vi "Read CellData.vi"(8 "error in":errorcluster, 11 "PAS Data in":refnum<class "PAS Data.lvclass">) -> (0 "error out":errorcluster, 2 "CellData":refnum<class "PAS Cell Data.lvclass">[](array[class]), 3 "PAS Data out":refnum<class "PAS Data.lvclass">)   [LabVIEW 2015, in "PAS Data.lvclass"]
doc: "Retrieve the data associated with the given cell."
uses:
  PAS Data.lvclass
  Cell/PAS Cell Data.lvclass
  PAS Data.lvclass/PAS Data.ctl
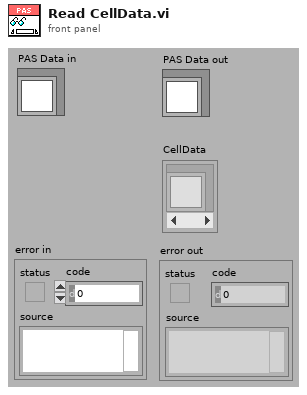
[diagram p1: front panel]
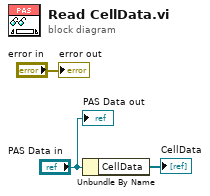
[diagram p0: block diagram]
diagram:
  n1 = Unbundle By Name("PAS Data in") -> ("CellData"=→"CellData":refnum<class "PAS Cell Data.lvclass">[])
  "error out" <- "error in"
  "PAS Data out" <- "PAS Data in"
